vi "generator_set_values.vi"(8 "error in (no error)":errorcluster, 9 "Amplitude (1.0 Vpp)":dbl=3.5 min=0.0 format="%#_13g", 10 "freq_value":dbl=100.0 min=0.0, 11 "UI in":T1) -> (0 "error out":errorcluster, 3 "UI_out":T1)   [LabVIEW 2017]
uses:
  ui.ctl
  classes/dc_power_supply/DC_power_supply.lvclass
  ui_buttons.ctl
  types/boc_type.ctl
  <instrlib>/Siglent SDG X Series/Siglent SDG X Series.lvlib
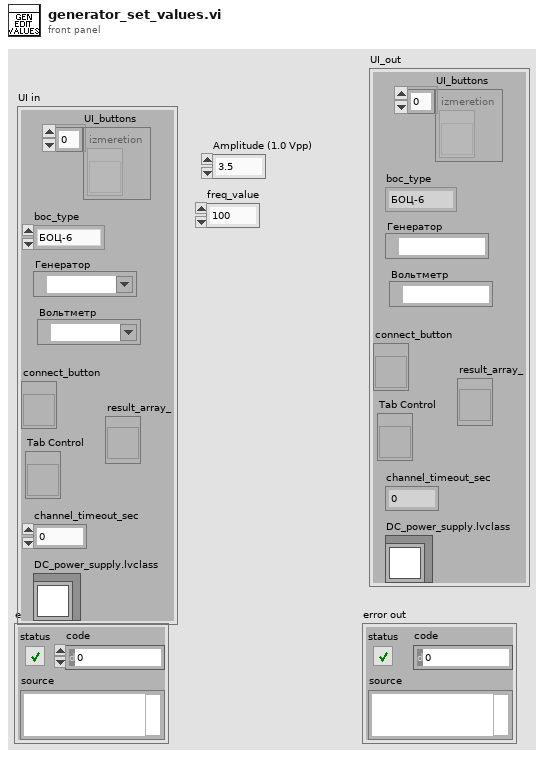
[diagram p1: front panel]
types:
  T1 = typedef "ui.ctl" = cluster{"UI_buttons":T2, "Tab Control":refnum<vi>, "connect_button":refnum<vi>, "generator":refnum<visa-resource-name>, "voltmetr":refnum<visa-resource-name>, "channel_timeout_sec":dbl, "boc_type":T3, "result_array_":refnum<vi>, "DC_power_supply.lvclass":refnum<class "DC_power_supply.lvclass">}
  T2 = typedef "ui_buttons.ctl" = refnum<vi>[]
  T3 = typedef "boc_type.ctl" = enum16{"БОЦ-6", "БОЦ-12"}
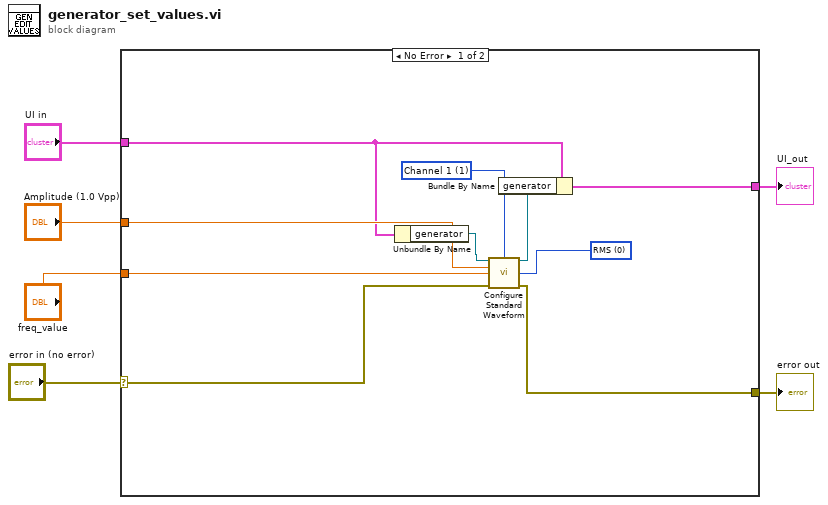
[diagram p0: block diagram]
diagram:
  n1 = case shown="No Error" "error in (no error)" {
    selector: "error in (no error)" -> [w8 w17]
    tunnel: "Amplitude (1.0 Vpp)" -> [w15 _]
    tunnel: "freq_value" -> [w14 _]
    tunnel: "UI in" -> [w10 w18]
    tunnel: [w12 w17] -> w3
    tunnel: [w9 w18] -> w2
    frame No Error {
      w7 = 1 items=["Channel 1"=1, "Channel 2"=2] ("Channel (1:Channel 1)")
      w16 = u16 0 items=["RMS", "pp", "dBm"] ("v-type")
      n2 = Unbundle By Name(w10) -> ("generator"=w13:refnum<visa-resource-name>)
      n3 = call <instrlib>:"Configure Standard Waveform.vi"("VISA resource name"=w13, "Channel (1:Channel 1)"=w7, "Amplitude (1.0 Vpp)"=w15, "Frequency (1000 Hz)"=w14, "v-type"=w16, "error in (no error)"=w8) -> ("VISA resource name out"=w11:refnum<visa-resource-name>, "error out"=w12:errorcluster)  [unwired: 8 in]
      n4 = Bundle By Name(cluster=w10, "generator"=w11) -> (w9:T1)
    }
    frame Error {
    }
  }
  "error out" <- w3
  "UI_out" <- w2
